vi "Initialize.vi"(6 "rmb?":bool, 8 "error in (no error)":errorcluster, 10 "max length":u8=5, 11 "recent user file":path) -> (0 "error out":errorcluster, 3 "[Data] Recent User out":refnum<class "[User] Recent Login.lvclass">)   [LabVIEW 2020, in "[User] Recent Login.lvclass"]
uses:
  [User] Recent Login.lvclass
  [User] Recent Login.lvclass/[User] Recent Login.ctl
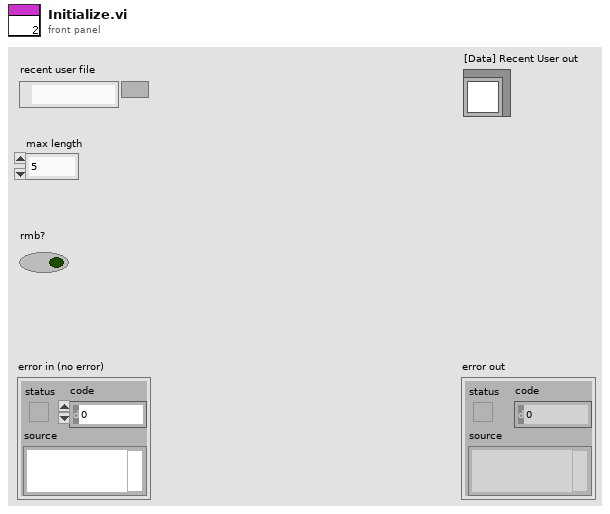
[diagram p1: front panel]
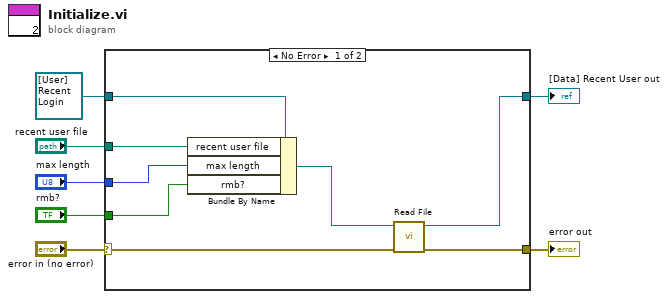
[diagram p0: block diagram]
diagram:
  n1 = case shown="No Error" "error in (no error)" {
    selector: "error in (no error)" -> [w13 w17]
    tunnel: [w10 w17] -> w6
    tunnel: [w11 w16] -> w4
    tunnel: refnum<class "[User] Recent Login.lvclass"> refnum ("[Data] Recent User in") -> [w15 w16]
    tunnel: "recent user file" -> [w14 _]
    tunnel: "max length" -> [w9 _]
    tunnel: "rmb?" -> [w8 _]
    frame No Error {
      n2 = Bundle By Name(cluster=w15, "recent user file"=w14, "max length"=w9, "rmb?"=w8) -> (w12:refnum<class "[User] Recent Login.lvclass">)
      n3 = call "Read File.vi"("error in (no error)"=w13, "[Data] Recent User in"=w12) -> ("error out"=w10:errorcluster, "[Data] Recent User out"=w11:refnum<class "[User] Recent Login.lvclass">)  [unwired: 8 in]
    }
    frame Error {
    }
  }
  "error out" <- w6
  "[Data] Recent User out" <- w4
